vi "Output DMA Engine.vi"(10 "Parameters":variant, 11 "Process":refnum<class "Process.lvclass">) -> ()   [LabVIEW 2019, in "FPGA Addon Engine.lvlib"]
uses:
  FPGA Addon Engine.lvlib
  <vilib>/NI/NIVS Inline Async API/_VS Inline Async API/Process/Process.lvclass
  Types/DMA Output References.ctl
  <vilib>/NI VeriStand/Custom Device Waveform API/Single Waveform Read (DBL)/Single Waveform Read (DBL).lvclass
  Types/DMA Output Refs.ctl
  Addon Shared/Data Type.ctl
  <vilib>/NI/NIVS Inline Async API/_VS Inline Async API/Process/Process.lvclass/Process.ctl
  <vilib>/Platform/TimedLoop/XDataNode/timing_clust.ctl
  <vilib>/Platform/TimedLoop/XDataNode/nitl_modes.ctl
  <vilib>/Platform/TimedLoop/XDataNode/wakeup.ctl
  <vilib>/NI/NIVS Inline Async API/_Data Access Engine/Access Type Classes/Write/Write.lvclass/Write.ctl
  <vilib>/NI/NIVS Inline Async API/_Data Access Engine/Data Access Engine/Methods/Write.Data.vi
  <vilib>/NI/NIVS Inline Async API/_VS Inline Async API/Process/Data Member Access/Read Data Access.vi
  <vilib>/NI/NIVS Inline Async API/_VS Inline Async API/Error Handling Process/SubVIs/Error.ConvertArray.vi
  <vilib>/NI/NIVS Inline Async API/_Data Access Engine/Access Type Classes/Write/Write.ProcessData.vi
  <vilib>/NI/NIVS Inline Async API/_Data Access Engine/Access Type Classes/Write/Write.Buffer.vi
  <vilib>/NI/NIVS Inline Async API/_Data Access Engine/Access Type Classes/Write/Write.Commit.vi
  <vilib>/Utility/SystemLogging/Write to System Log.vi
  <vilib>/NI/NIVS Inline Async API/_Data Access Engine/Data Access Engine/Methods/Write.Lookup.vi
  <vilib>/FPGAPlugInAG/Dynamic/niLvFpga_Close_Dynamic.vi
  <vilib>/NI VeriStand/Custom Device Waveform API/Single Waveform Read (DBL)/NI VeriStand - Close Single Waveform Read Session (DBL).vi
  <vilib>/NI/NIVS Inline Async API/_Data Access Engine/Data Access Engine/Data Access Engine.lvclass
  <vilib>/Platform/TimedLoop/XDataNode/XDataNode.xnode
  <vilib>/rvi/interface/nirviCloseFPGA/nirviCloseFPGA.xnode
  <vilib>/NI VeriStand/Custom Device Waveform API/NI_VS Custom Device Waveform API.lvlib
  <vilib>/Platform/TimedLoop/XDataNode/XDNodeRunTimeDep.lvlib
  Addon Shared/FPGA Addon Shared.lvlib
panel:
  out "error out":errorcluster
  in  "error in (no error)":errorcluster
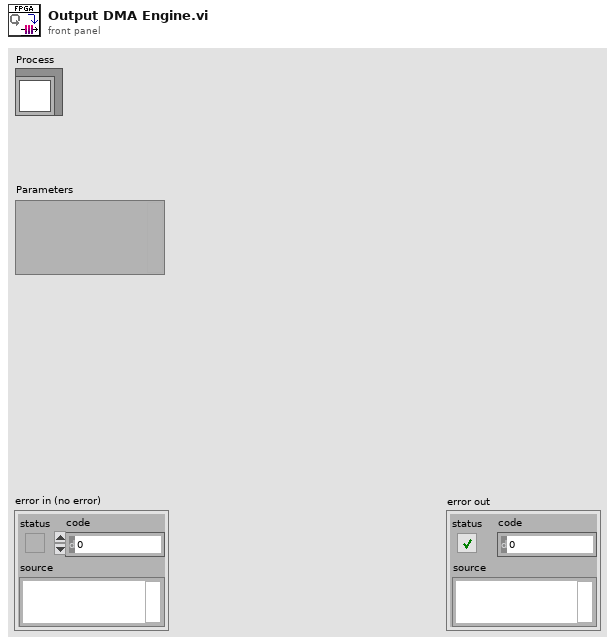
[diagram p1: front panel]
types:
  T1 = typedef "FPGA Addon Engine.lvlib/DMA Output References.ctl" = cluster{"Addon Name":string, "Waveforms":refnum<class "Single Waveform Read (DBL).lvclass">[], "DMA Name":string, "Refs":T2}
  T2 = typedef "FPGA Addon Engine.lvlib/DMA Output Refs.ctl" = cluster{"Data Type":T3, "DMA_SGL":refnum<k20>, "DMA_U64":refnum<k20>, "DMA_I64":refnum<k20>, "DMA_FXP+/-32.8":refnum<k20>, "DMA_FXP+/-64.32":refnum<k20>, "DMA_U32":refnum<k20>, "DMA_U16":refnum<k20>, "DMA_U8":refnum<k20>, "DMA_I32":refnum<k20>, "DMA_I16":refnum<k20>, "DMA_I8":refnum<k20>, "DMA_FXP+/-32.16":refnum<k20>}
  T3 = typedef "FPGA Addon Shared.lvlib/Data Type.ctl" = enum8{"<Null>", "I8", "I16", "I32", "I64", "U8", "U16", "U32", "U64", "SGL", "Boolean", "Analog PWM In Settings", "Analog PWM In", "Digital PWM In Settings", "Digital PWM In", "Digital PWM Out", "Sine Out", "FXP+/-24.5", "FXP+/-16.5", "FXP+/-32.8", "FXP+/-64.32", "FXP+/-16.7", "FXP+/-20.5", "FXP+/-27.5", "FXP+/-32.16", "FXP +16.3", "FXP +18.3", "Digital Static In", "Digital Static Out", "Digital Static In Settings", "Digital WSS Out", "Quad Encoder Settings", "Quad Encoder In"}
  T4 = typedef "Data Access Engine.lvlib/Data Access Engine.lvclass/Write.DVR.ctl" = refnum<data-value>
  T5 = typedef "XDNodeRunTimeDep.lvlib/timing_clust.ctl" = cluster{"Expected End [f-1]":u64, "Actual End [f-1]":u64, "Finished Late? [f-1]":bool, "Expected End [i-1]":u64, "Actual End [i-1]":u64, "Finished Late? [i-1]":bool, "Expected Start [i]":u64, "Actual Start [i]":u64, "Expected Start [f]":u64, "Actual Start [f]":u64, "Source Name":string, "Structure Name":string, "Period":i64, "Deadline":i64, "Offset":i64, "Start":i64, "Priority":i32, "Timeout":i32, "Mode":T6, "Wakeup Reason":T7, "Error":errorcluster, "Source Type":string, "Secondary Source Type":string, "Global End Time":u64, "Global Start Time":u64, "Frame Duration":u64, "Iteration Duration":u64, "Assigned CPU":i32, "I/O Scan Engine Mode":u32}
  T6 = typedef "XDNodeRunTimeDep.lvlib/nitl_modes.ctl" = enum32{"No Change", "Process missed periods, maintain original phase", "Discard missed periods, maintain original phase", "Process missed periods, ignore original phase", "Discard missed periods, ignore original phase"}
  T7 = typedef "XDNodeRunTimeDep.lvlib/wakeup.ctl" = enum32{"Normal", "Aborted", "Asynchronous wakeup", "Timing source error", "Timed loop error", "Timeout"}
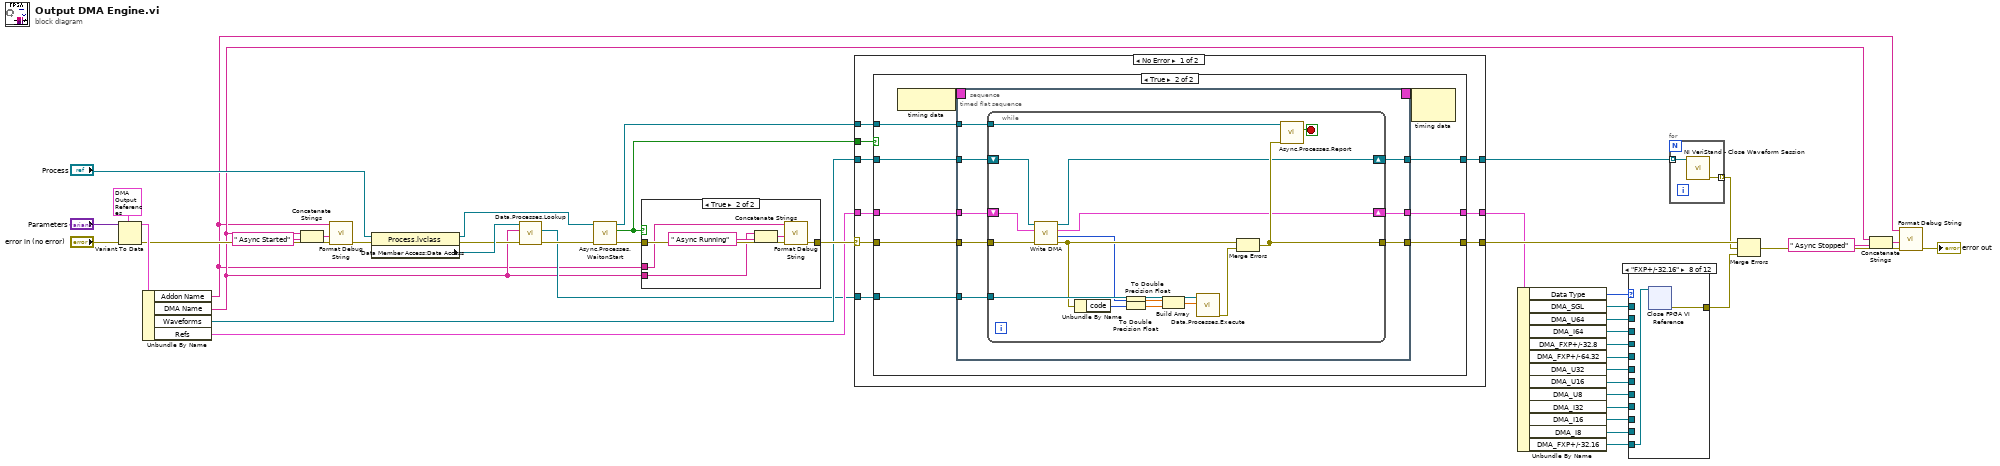
[diagram p0: block diagram]
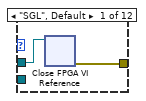
[diagram p2: hidden frame]
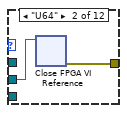
[diagram p3: hidden frame]
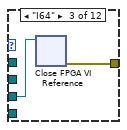
[diagram p4: hidden frame]
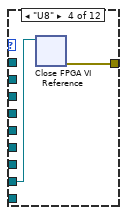
[diagram p5: hidden frame]
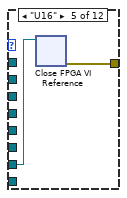
[diagram p6: hidden frame]
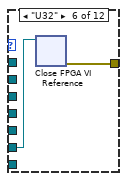
[diagram p7: hidden frame]
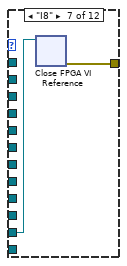
[diagram p8: hidden frame]
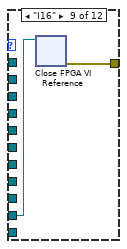
[diagram p9: hidden frame]
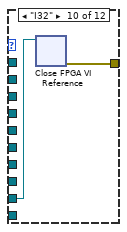
[diagram p10: hidden frame]
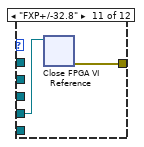
[diagram p11: hidden frame]
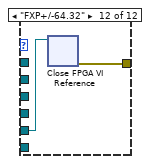
[diagram p12: hidden frame]
diagram:
  n1 = Variant To Data(error in="error in (no error)", type=T1 {"Addon Name"="", "Waveforms"=[], "DMA Name"="", "Refs"={"Data Type"=enum."I32", "DMA_SGL"=refnum, "DMA_U64"=refnum, "DMA_I64"=refnum, "DMA_FXP+/-32.8"=refnum, "DMA_FXP+/-64.32"=refnum, "DMA_U32"=refnum, "DMA_U16"=refnum, "DMA_U8"=refnum, "DMA_I32"=refnum, "DMA_I16"=refnum, "DMA_I8"=refnum, "DMA_FXP+/-32.16"=refnum}} ("Parameters"), Variant="Parameters") -> (data=w25:T1, error out=w23:errorcluster)
  n2 = Unbundle By Name(w25) -> ("Addon Name"=w1:string, "DMA Name"=w21:string, "Waveforms"=w37:refnum<class "Single Waveform Read (DBL).lvclass">[], "Refs"=w36:T2)
  n3 = Concatenate Strings(w21, " Async Started" ("string")) -> (w19:string)
  n4 = call "Format Debug String.vi"("error in (no error)"=w23, "State"=w19, "Name"=w1) -> ("error out"=w22:errorcluster)  [unwired: 8 in]
  n5 = property class="Process.lvclass"(reference="Process", error in=w22) -> (reference out=w31:refnum<class "Process.lvclass">, error out=w29:errorcluster, "Data Member Access:Data Access"=w30:refnum<class "Data Access Engine.lvclass">)
  n6 = call-poly <vilib>:"Data.Processes.Lookup.vi"("error in (no error)"=w29, "Name"=w21, "Data Access API in"=w30) -> ("error out"=w28:errorcluster, "Ref"=w27:T4)  [unwired: 5 in, 2 out]
  n7 = call <vilib>:"Async.Processes.WaitonStart.vi"("error in (no error)"=w28, "Process"=w31) -> ("error out"=w34:errorcluster, "Execute"=w35:bool, "Process out"=w33:refnum<class "Process.lvclass">)  [unwired: 7 in]
  n8 = case shown="True" w35 {
    tunnel: w21 -> [_ w47]
    tunnel: w34 -> [w45 w49]
    tunnel: [w45 w48] -> w40
    tunnel: w1 -> [_ w46]
    frame False {
    }
    frame True {
      n9 = Concatenate Strings(w47, " Async Running" ("string")) -> (w50:string)
      n10 = call "Format Debug String.vi"("error in (no error)"=w49, "State"=w50, "Name"=w46) -> ("error out"=w48:errorcluster)  [unwired: 8 in]
    }
  }
  n11 = case shown="No Error" w40 {
    selector: w40 -> [w57 w110]
    tunnel: [w60 w112] -> w43
    tunnel: [w59 w110] -> w42
    tunnel: w33 -> [w58 _]
    tunnel: w35 -> [w56 _]
    tunnel: [w55 w111] -> w41
    tunnel: w27 -> [w54 _]
    tunnel: w37 -> [w53 w112]
    tunnel: w36 -> [w52 w111]
    frame No Error {
      n12 = case shown="True" w56 {
        tunnel: [w61 w73] -> w60
        tunnel: [w63 w72] -> w59
        tunnel: w58 -> [_ w71]
        tunnel: w57 -> [w63 w70]
        tunnel: [w62 w69] -> w55
        tunnel: w54 -> [_ w68]
        tunnel: w53 -> [w61 w67]
        tunnel: w52 -> [w62 w66]
        frame False {
        }
        frame True {
          n13 = node-c288() -> (w65:T5)
          n14 = timed-sequence {
            timing: w65 -> [_]
            timing-out: [_] -> w64
            tunnel: [w81] -> w73
            tunnel: [w80] -> w72
            tunnel: w71 -> [w79]
            tunnel: w70 -> [w78]
            tunnel: [w77] -> w69
            tunnel: w68 -> [w76]
            tunnel: w67 -> [w75]
            tunnel: w66 -> [w74]
            n15 = timed-flat-sequence {
              tunnel: [w89] -> w81
              tunnel: [w88] -> w80
              tunnel: w79 -> [w87]
              tunnel: w78 -> [w86]
              tunnel: [w85] -> w77
              tunnel: w76 -> [w84]
              tunnel: w75 -> [w83]
              tunnel: w74 -> [w82]
              n16 = while {
                tunnel: w87 -> [w105]
                tunnel: w84 -> [w103]
                shift-right: [w95] -> w85
                shift-left: w82 -> [w96]
                shift-right: [w100] -> w89
                shift-left: w83 -> [w97]
                tunnel: w86 -> [w99]
                tunnel: [w101] -> w88
                stop <- w94 stop-if-true
                n17 = call "Write DMA.vi"("error in (no error)"=w99, "Refs"=w96, "Waveform Refs"=w97) -> ("error out"=w98:errorcluster, "Empty Elements Remaining"=w91:u32, "Refs out"=w95:T2, "Waveform Refs"=w100:refnum<class "Single Waveform Read (DBL).lvclass">[])  [unwired: 5 in]
                n18 = Unbundle By Name(w98) -> ("code"=w93:i32)
                n19 = To Double Precision Float(number=w91) -> (double precision float=w90:dbl)
                n20 = To Double Precision Float(number=w93) -> (double precision float=w92:dbl)
                n21 = Build Array(w90, w92) -> (w104:dbl[])
                n22 = call-poly <vilib>:"Data.Processes.Execute.vi"("Values"=w104, "Ref"=w103) -> ("error out"=w102:errorcluster)  [unwired: 9 in]
                n23 = Merge Errors(w98, w102) -> (w101:errorcluster)
                n24 = call <vilib>:"Async.Processes.Report.vi"("Error"=w101, "Process in"=w105) -> ("Stop"=w94:bool)  [unwired: 8 in, 1 out]
              }
            }
          }
          n25 = node-c288(w64) -> ()  [unwired: 1 out]
        }
      }
    }
    frame Error {
    }
  }
  n26 = Unbundle By Name(w41) -> ("Data Type"=w17:T3, "DMA_SGL"=w16:refnum<k20>, "DMA_U64"=w15:refnum<k20>, "DMA_I64"=w14:refnum<k20>, "DMA_FXP+/-32.8"=w12:refnum<k20>, "DMA_FXP+/-64.32"=w11:refnum<k20>, "DMA_U32"=w10:refnum<k20>, "DMA_U16"=w9:refnum<k20>, "DMA_U8"=w8:refnum<k20>, "DMA_I32"=w7:refnum<k20>, "DMA_I16"=w6:refnum<k20>, "DMA_I8"=w5:refnum<k20>, "DMA_FXP+/-32.16"=w4:refnum<k20>)
  n27 = case shown="\"FXP+/-32.16\"" w17 {
    tunnel: [w114 w116 w118 w120 w122 w124 w126 w128 w130 w132 w134 w136] -> w13
    tunnel: w16 -> [w113 _ _ _ _ _ _ _ _ _ _ _]
    tunnel: w15 -> [_ w115 _ _ _ _ _ _ _ _ _ _]
    tunnel: w14 -> [_ _ w117 _ _ _ _ _ _ _ _ _]
    tunnel: w12 -> [_ _ _ _ _ _ _ _ _ _ w133 _]
    tunnel: w11 -> [_ _ _ _ _ _ _ _ _ _ _ w135]
    tunnel: w10 -> [_ _ _ _ _ w123 _ _ _ _ _ _]
    tunnel: w9 -> [_ _ _ _ w121 _ _ _ _ _ _ _]
    tunnel: w8 -> [_ _ _ w119 _ _ _ _ _ _ _ _]
    tunnel: w7 -> [_ _ _ _ _ _ _ _ _ w131 _ _]
    tunnel: w6 -> [_ _ _ _ _ _ _ _ w129 _ _ _]
    tunnel: w5 -> [_ _ _ _ _ _ w125 _ _ _ _ _]
    tunnel: w4 -> [_ _ _ _ _ _ _ w127 _ _ _ _]
    frame "SGL", Default {
      n28 = xnode "Close FPGA VI Reference"("FPGA VI Reference In"=w113) -> ("error out"=w114:errorcluster)  [unwired: 1 in]
    }
    frame "U64" {
      n29 = xnode "Close FPGA VI Reference"("FPGA VI Reference In"=w115) -> ("error out"=w116:errorcluster)  [unwired: 1 in]
    }
    frame "I64" {
      n30 = xnode "Close FPGA VI Reference"("FPGA VI Reference In"=w117) -> ("error out"=w118:errorcluster)  [unwired: 1 in]
    }
    frame "U8" {
      n31 = xnode "Close FPGA VI Reference"("FPGA VI Reference In"=w119) -> ("error out"=w120:errorcluster)  [unwired: 1 in]
    }
    frame "U16" {
      n32 = xnode "Close FPGA VI Reference"("FPGA VI Reference In"=w121) -> ("error out"=w122:errorcluster)  [unwired: 1 in]
    }
    frame "U32" {
      n33 = xnode "Close FPGA VI Reference"("FPGA VI Reference In"=w123) -> ("error out"=w124:errorcluster)  [unwired: 1 in]
    }
    frame "I8" {
      n34 = xnode "Close FPGA VI Reference"("FPGA VI Reference In"=w125) -> ("error out"=w126:errorcluster)  [unwired: 1 in]
    }
    frame "FXP+/-32.16" {
      n35 = xnode "Close FPGA VI Reference"("FPGA VI Reference In"=w127) -> ("error out"=w128:errorcluster)  [unwired: 1 in]
    }
    frame "I16" {
      n36 = xnode "Close FPGA VI Reference"("FPGA VI Reference In"=w129) -> ("error out"=w130:errorcluster)  [unwired: 1 in]
    }
    frame "I32" {
      n37 = xnode "Close FPGA VI Reference"("FPGA VI Reference In"=w131) -> ("error out"=w132:errorcluster)  [unwired: 1 in]
    }
    frame "FXP+/-32.8" {
      n38 = xnode "Close FPGA VI Reference"("FPGA VI Reference In"=w133) -> ("error out"=w134:errorcluster)  [unwired: 1 in]
    }
    frame "FXP+/-64.32" {
      n39 = xnode "Close FPGA VI Reference"("FPGA VI Reference In"=w135) -> ("error out"=w136:errorcluster)  [unwired: 1 in]
    }
  }
  n40 = for {
    tunnel: w43 -> [w138] mode=indexing
    tunnel: [w137] -> w18 mode=indexing
    n41 = call-poly <vilib>:"NI VeriStand - Close Waveform Session.vi"("Single Waveform Read Session (DBL)"=w138) -> ("error out"=w137:errorcluster)  [unwired: 10 in]
  }
  n42 = Merge Errors(w42, w18, w13) -> (w44:errorcluster)
  n43 = Concatenate Strings(w21, " Async Stopped" ("string")) -> (w2:string)
  n44 = call "Format Debug String.vi"("error in (no error)"=w44, "State"=w2, "Name"=w1) -> ("error out"=→"error out":errorcluster)  [unwired: 8 in]
